vi "Get Server State Ref.vi"(11 "Template Server in":refnum<class "OCV.lvclass">) -> (2 "Server State Ref":refnum<data-value>, 3 "Template Server out":refnum<class "OCV.lvclass">)   [LabVIEW 2019, in "OCV.lvlib" / "OCV.lvclass"]
uses:
  OCV.lvclass
  typeDefs/Server State Data.ctl
  OCV.lvclass/OCV.ctl
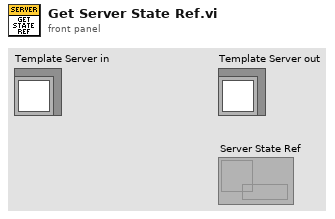
[diagram p1: front panel]
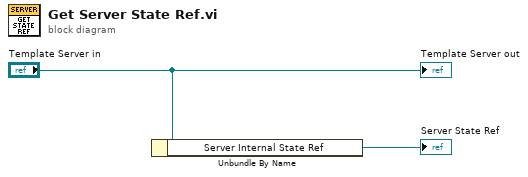
[diagram p0: block diagram]
diagram:
  n1 = Unbundle By Name("Template Server in") -> ("Server Internal State Ref"=→"Server State Ref":refnum<data-value>)
  "Template Server out" <- "Template Server in"
